vi "dice.vi"() -> (3 "y":dbl=5.0)   [LabVIEW 2014]
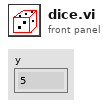
[diagram p1: front panel]
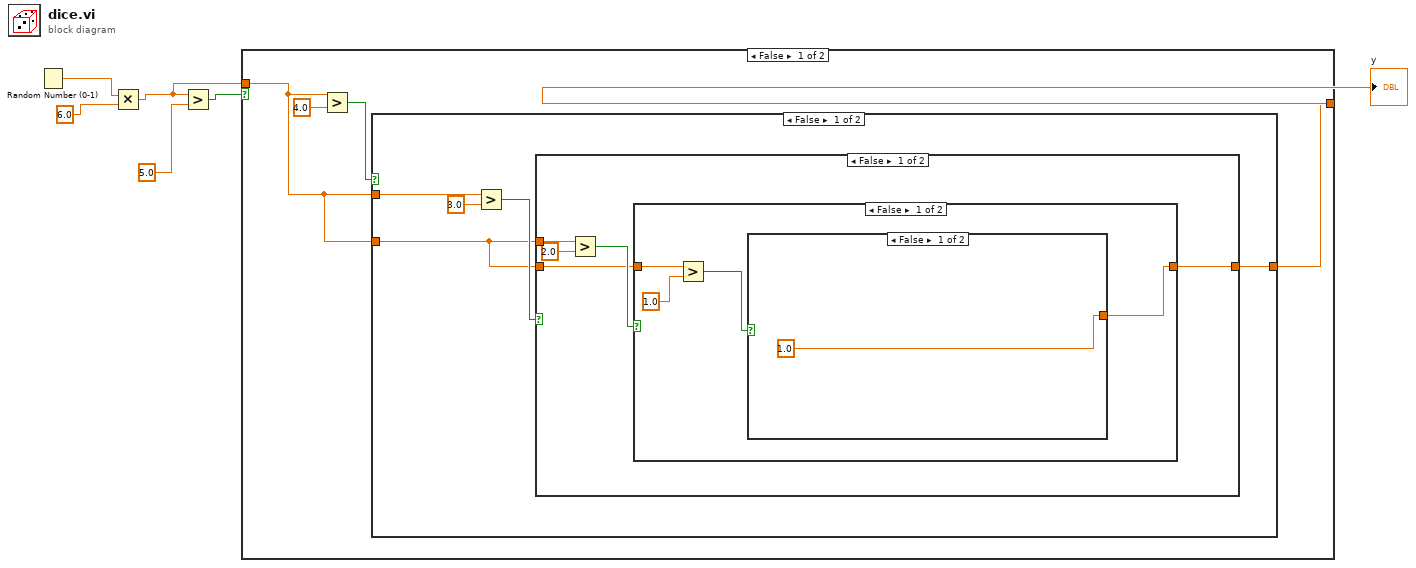
[diagram p0: block diagram]
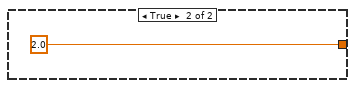
[diagram p2: hidden frame]
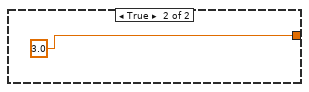
[diagram p3: hidden frame]
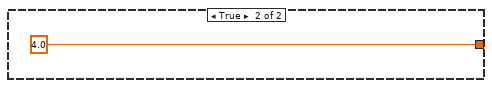
[diagram p4: hidden frame]
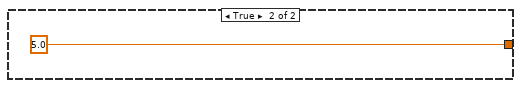
[diagram p5: hidden frame]
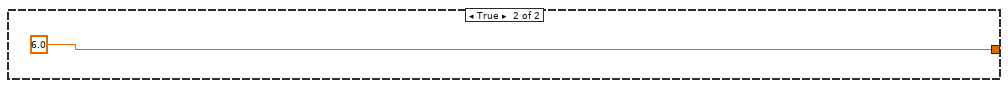
[diagram p6: hidden frame]
diagram:
  n1 = Random Number (0-1)() -> (number: 0 to 1=w6:dbl)
  n2 = Multiply(x=w6, y=6.0 ("number (0 to 1)")) -> (x*y=w1:dbl)
  n3 = Greater?(x=w1, y=5.0) -> (0:w3:bool)
  n4 = case shown="False" w3 {
    tunnel: [w8 6.0 ("y")] -> w2
    tunnel: w1 -> [w7 _]
    frame False {
      n5 = Greater?(x=w7, y=4.0) -> (0:w9:bool)
      n6 = case shown="False" w9 {
        tunnel: [w12 5.0 ("y")] -> w8
        tunnel: w7 -> [w15 _]
        tunnel: w7 -> [w11 _]
        frame False {
          n7 = Greater?(x=w15, y=3.0) -> (0:w13:bool)
          n8 = case shown="False" w13 {
            tunnel: [w17 4.0 ("y")] -> w12
            tunnel: w11 -> [w20 _]
            tunnel: w11 -> [w16 _]
            frame False {
              n9 = Greater?(x=w20, y=2.0) -> (0:w18:bool)
              n10 = case shown="False" w18 {
                tunnel: [w21 3.0 ("y")] -> w17
                tunnel: w16 -> [w24 _]
                frame False {
                  n11 = Greater?(x=w24, y=1.0) -> (0:w22:bool)
                  n12 = case shown="False" w22 {
                    tunnel: [1.0 ("y") 2.0 ("y")] -> w21
                    frame False {
                    }
                    frame True {
                    }
                  }
                }
                frame True {
                }
              }
            }
            frame True {
            }
          }
        }
        frame True {
        }
      }
    }
    frame True {
    }
  }
  "y" <- w2
